vi "StartSequenceAcq.vi"(8 "error in (no error)":errorcluster, 11 "Config In":T1 {"Hardware Configuration"."Lasers Configuration"."SettingValues"."785 Power" format="%.1f"; "Hardware Configuration"."Lasers Configuration"."SettingValues"."647 Power" format="%.1f"; "Hardware Configuration"."Lasers Configuration"."SettingValues"."561 Power" format="%.1f"}) -> (0 "error out":errorcluster, 3 "Config Out":T1 {"Hardware Configuration"."Lasers Configuration"."SettingValues"."785 Power" format="%.1f"; "Hardware Configuration"."Lasers Configuration"."SettingValues"."647 Power" format="%.1f"; "Hardware Configuration"."Lasers Configuration"."SettingValues"."561 Power" format="%.1f"})   [LabVIEW 2019]
uses:
  Settings/System Running Settings.ctl
  Support/Hardware Configuration.ctl
  Support/Camera Configuration.ctl
  C:/RM21-MMicrosopeSource/HardwareAdapter/Camera/Dependencies/PVCamNET.dll
  Dependencies/PVCamNET.dll
  <vilib>/vision/Image Controls.llb/IMAQ Image.ctl
  C:/RM21-MMicrosopeSource/HardwareAdapter/Lasers/Dependencies/Oxxius_Boxx.dll
  Lasers/Dependencies/Oxxius_Boxx.dll
  Logging/Logging Configuration.ctl
  Controls/DeviceStatusCtl.ctl
  Controls/CallBack Refs.ctl
  Global.vi
  Logging/Logging.lvlib
  Settings/Settings.lvlib
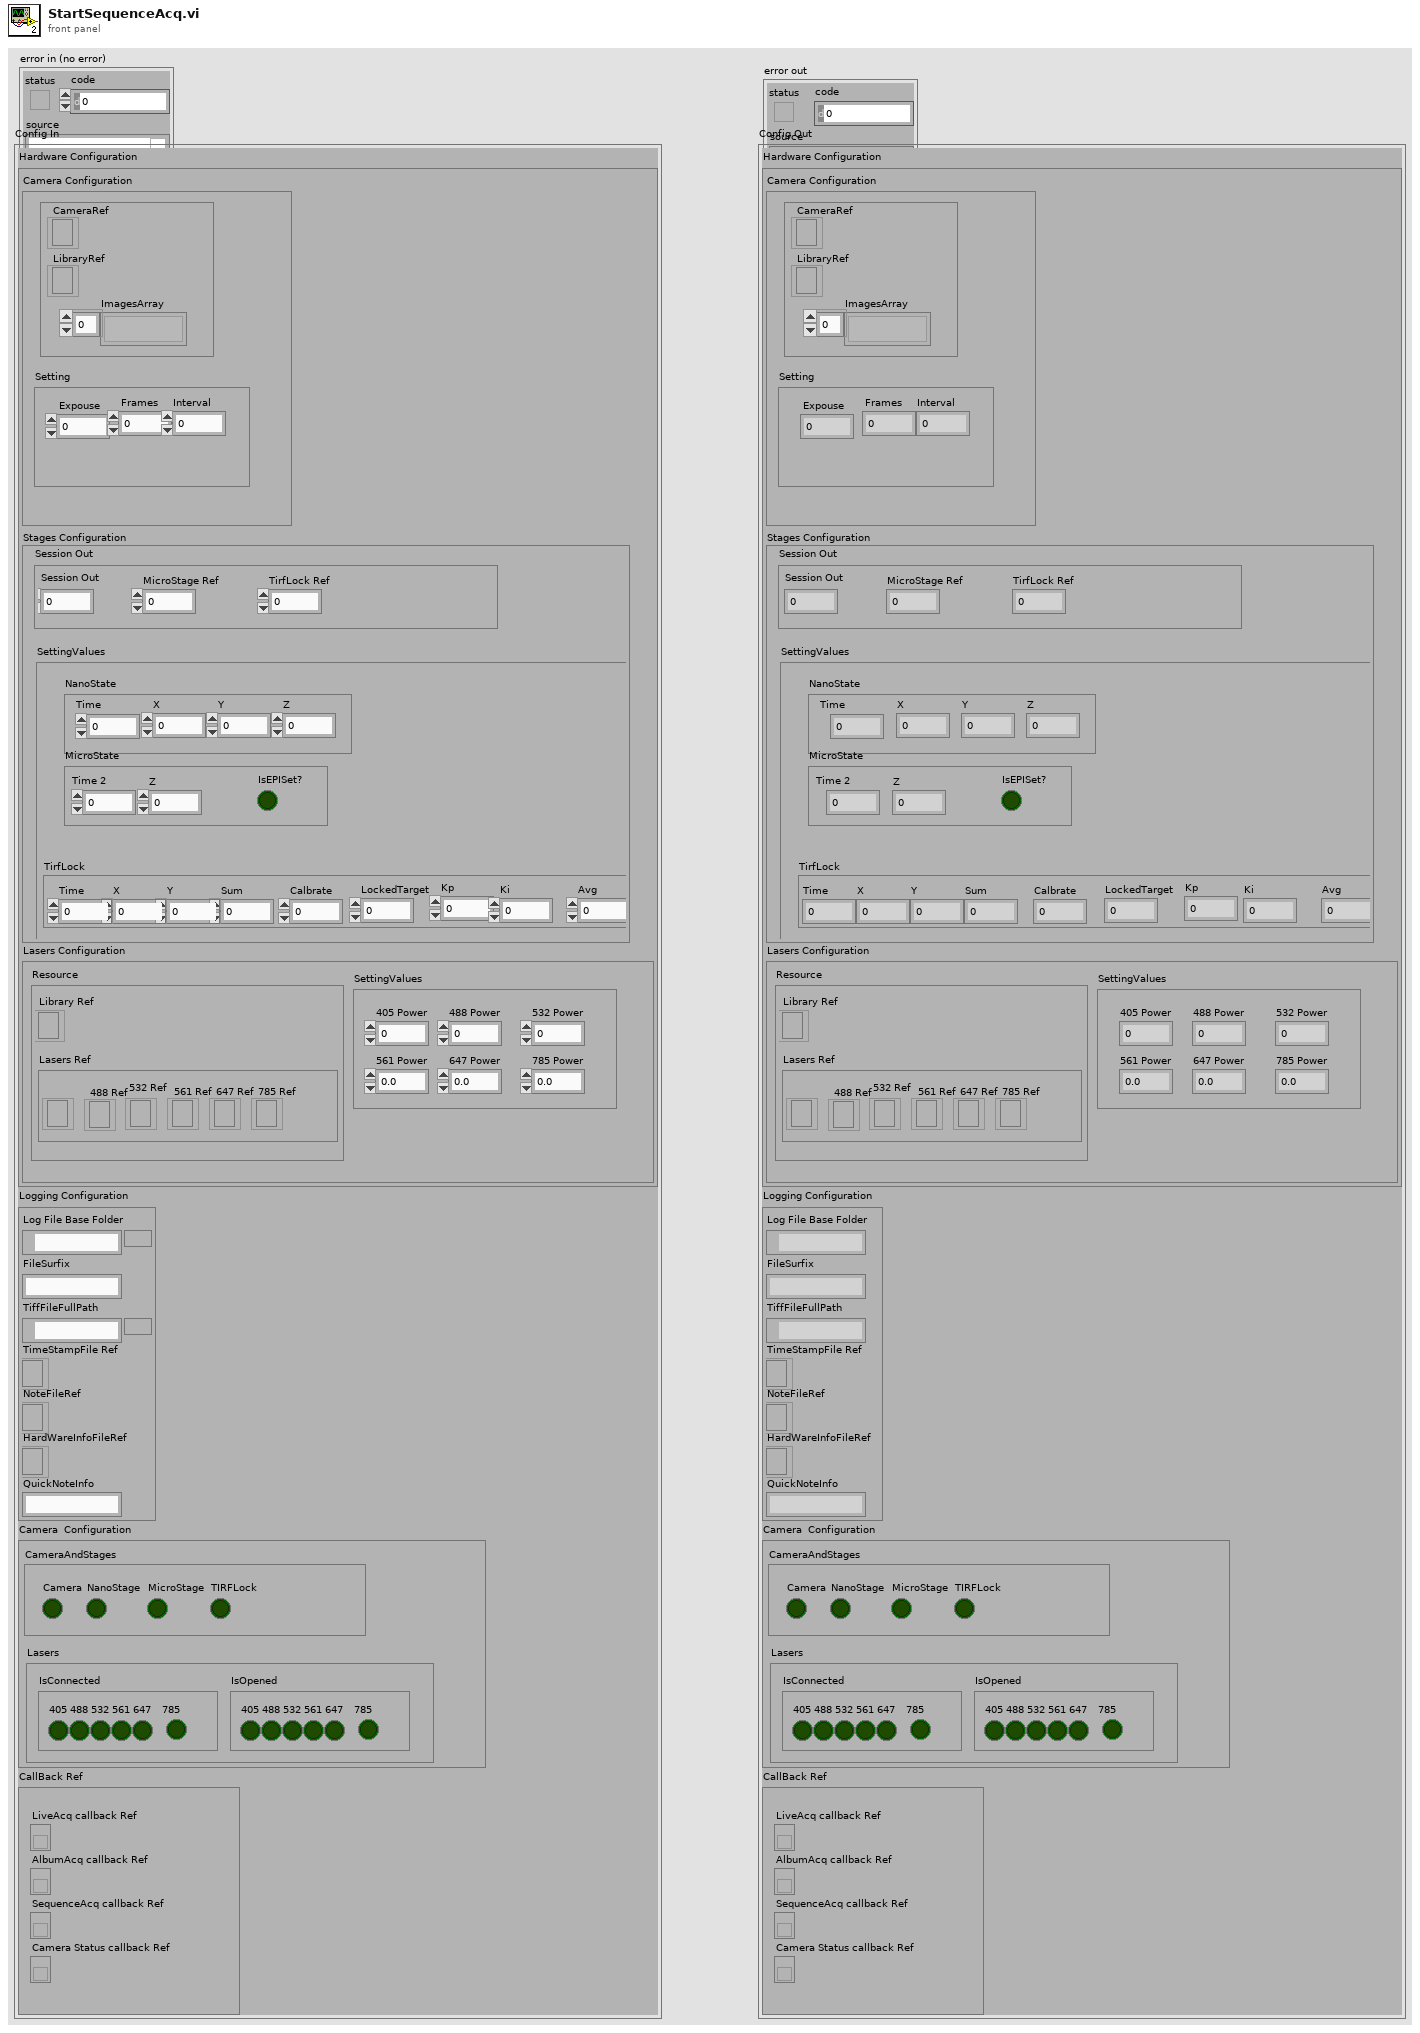
[diagram p1: front panel]
types:
  T1 = typedef "Settings.lvlib/System Running Settings.ctl" = cluster{"Hardware Configuration":T2, "Logging Configuration":T5, "HardWare Status":cluster{"CameraAndStages":T6, "Lasers":cluster{"IsConnected":cluster{"405":bool, "488":bool, "532":bool, "561":bool, "647":bool, "785":bool}, "IsOpened":cluster{"405":bool, "488":bool, "532":bool, "561":bool, "647":bool, "785":bool}}}, "CallBack Ref":T7}
  T2 = typedef "Hardware Configuration.ctl" = cluster{"Camera Configuration":T3, "Stages Configuration":cluster{"Resource":cluster{"NanoStage Ref":i32, "MicroStage Ref":i32, "TirfLock Ref":i32}, "SettingValues":cluster{"NanoState":cluster{"Time":dbl, "X":dbl, "Y":dbl, "Z":dbl}, "MicroState":cluster{"Time 2":dbl, "Z":dbl, "IsEPISet?":bool}, "TirfLock":cluster{"Time":dbl, "X":dbl, "Y":dbl, "Sum":dbl, "Calbrate":dbl, "LockedTarget":dbl, "Kp":dbl, "Ki":dbl, "Avg":dbl}}}, "Lasers Configuration":cluster{"SettingValues":cluster{"405 Power":sgl, "488 Power":sgl, "532 Power":sgl, "561 Power":sgl, "647 Power":sgl, "785 Power":sgl}, "Resource":cluster{"Library Ref":refnum<k24>, "Lasers Ref":cluster{"405 Ref":refnum<k24>, "488 Ref":refnum<k24>, "532 Ref":refnum<k24>, "561 Ref":refnum<k24>, "647 Ref":refnum<k24>, "785 Ref":refnum<k24>}}}}
  T3 = typedef "Camera Configuration.ctl" = cluster{"Setting":cluster{"Expouse":dbl, "Frames":dbl, "Interval":dbl}, "Resource":cluster{"CameraRef":refnum<k24>, "LibraryRef":refnum<k24>, "ImagesArray":T4[]}}
  T4 = typedef "IMAQ Image.ctl" = refnum<image>
  T5 = typedef "Logging.lvlib/Logging Configuration.ctl" = cluster{"Log File Base Folder":path, "FileSurfix":string, "TiffFileFullPath":path, "TimeStampFile Ref":refnum<file>, "NoteFileRef":refnum<file>, "HardWareInfoFileRef":refnum<file>, "QuickNoteInfo":string}
  T6 = typedef "DeviceStatusCtl.ctl" = cluster{"Camera":bool, "NanoStage":bool, "MicroStage":bool, "TIRFLock":bool}
  T7 = typedef "CallBack Refs.ctl" = cluster{"LiveAcq callback Ref":refnum<k27>, "AlbumAcq callback Ref":refnum<k27>, "SequenceAcq callback Ref":refnum<k27>, "Camera Status callback Ref":refnum<k27>}
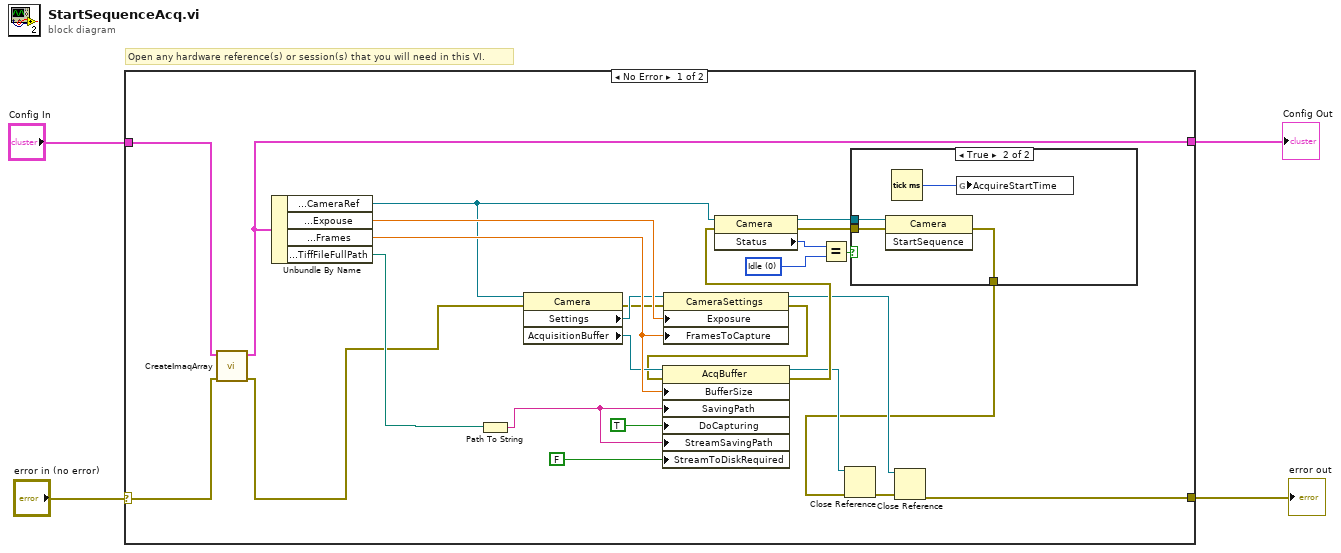
[diagram p0: block diagram]
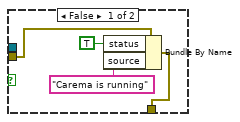
[diagram p2: hidden frame]
diagram:
  # "Open any hardware reference(s) or session(s) that you will need in this VI."
  n1 = case shown="No Error" "error in (no error)" {
    selector: "error in (no error)" -> [w12 w39]
    tunnel: [w6 w39] -> w3
    tunnel: "Config In" -> [w11 w40]
    tunnel: [w10 w40] -> w1
    frame No Error {
      w23 = 0 items=["Idle", "Capturing"] ("Status")
      n2 = call "CreateImaqArray.vi"("error in (no error)"=w12, "Config"=w11) -> ("error in (no error) 2"=w13:errorcluster, "Config 2"=w10:T1)  [unwired: 8 in]
      n3 = Unbundle By Name(w10) -> ("Hardware Configuration.Camera Configuration.Resource.CameraRef"=w28:refnum<k24>, "Hardware Configuration.Camera Configuration.Setting.Expouse"=w30:dbl, "Hardware Configuration.Camera Configuration.Setting.Frames"=w29:dbl, "Logging Configuration.TiffFileFullPath"=w27:path)
      n4 = Path To String(path=w27) -> (string=w15:string)
      n5 = property class="Camera"(reference=w28, error in=w13) -> (error out=w25:errorcluster, "Settings"=w26:refnum<k24>, "AcquisitionBuffer"=w24:refnum<k24>)  [unwired: 1 out]
      n6 = property class="CameraSettings"(reference=w26, error in=w25, "Exposure"=w30, "FramesToCapture"=w29) -> (reference out=w7:refnum<k24>, error out=w18:errorcluster)
      n7 = property class="AcqBuffer"(reference=w24, error in=w18, "BufferSize"=w29, "SavingPath"=w15, "DoCapturing"=TRUE, "StreamSavingPath"=w15, "StreamToDiskRequired"=FALSE) -> (reference out=w9:refnum<k24>, error out=w17:errorcluster)
      n8 = property class="Camera"(reference=w28, error in=w17) -> (reference out=w20:refnum<k24>, error out=w19:errorcluster, "Status"=w22:i32)
      n9 = Equal?(x=w22, y=w23) -> (x = y?=w21:bool)
      n10 = case shown="True" w21 {
        tunnel: [w31 w38] -> w5
        tunnel: w20 -> [_ w37]
        tunnel: w19 -> [w32 w36]
        frame False {
          n11 = Bundle By Name(cluster=w32, "status"=TRUE, "source"="Carema is running") -> (w31:errorcluster)
        }
        frame True {
          n12 = invoke class="Camera" method="StartSequence"(reference=w37, error in=w36) -> (error out=w38:errorcluster)  [unwired: 1 in, 2 out]
          n13 = Tick Count (ms)() -> (millisecond timer value=w35:u32)
          n14 = global write "Global.vi" "AcquireStartTime"(w35) -> ()
        }
      }
      n15 = Close Reference(reference=w9, error in (no error)=w5) -> (error out=w8:errorcluster)
      n16 = Close Reference(reference=w7, error in (no error)=w8) -> (error out=w6:errorcluster)
    }
    frame Error {
    }
  }
  "error out" <- w3
  "Config Out" <- w1
